vi "Main.vi"(11 "Module Admin":refnum<class "Delacor_lib_QMH_Cloneable Module Admin.lvclass">) -> ()   [LabVIEW 2024, in "cameraV1.lvlib"]
doc: "This template is based off of the Queued Message Handler design pattern and the Queued Message Handler project template that ships with LabVIEW.\n\nThe main difference is that the queue is private to this module and communication between modules is performed via Broadcast and Request events.\n\nRequest events are wrapped in public API methods and are handled in the Event Handling Loop (EHL) of this VI. Any module can register for Broadcast events sent by this module. The EHL generates messages based on user interface actions.\n\nThe Message Handling Loop (MHL) processes messages generated by the EHL, or by other messages. The messages are string values, so new messages can be added easily to the Message Cases case structure in the MHL. Each message cluster can also provide an optional value for Message Data, which is a variant that can be converted to whatever message-specific data is required.\n_____\nBased on DQMH Dev Tools: Project Template 7.1.0.1503."
uses:
  cameraV1.lvlib
  <vilib>/Delacor/Delacor QMH/Libraries/Cloneable Module Admin_class/Delacor_lib_QMH_Cloneable Module Admin.lvclass
  Controls/camera module state.ctl
  Controls/state.ctl
  Module Data--cluster.ctl
  <vilib>/Delacor/Delacor QMH/Libraries/Message Queue_class/Delacor_lib_QMH_Message Queue.lvclass/Delacor_lib_QMH_Message Queue.ctl
  <vilib>/Delacor/Delacor QMH/Libraries/Cloneable Module Admin_class/Delacor_lib_QMH_Cloneable Module Admin.lvclass/Delacor_lib_QMH_Cloneable Module Admin.ctl
  Stop Argument--cluster.ctl
  <vilib>/Delacor/Delacor QMH/Libraries/Module Admin_class/Delacor_lib_QMH_Module Admin.lvclass/Delacor_lib_QMH_Module Admin.ctl
  connect Argument--cluster.ctl
  Send_Command Argument--cluster.ctl
  Controls/commands 1.ctl
  Send_Command (Reply Payload)--cluster.ctl
  Cam Image Response Argument--cluster.ctl
  <vilib>/Utility/miscctls.llb/LVPointTypeDef.ctl
  <vilib>/Delacor/Delacor QMH/Libraries/Message Queue_class/Delacor_lib_QMH_Enqueue Message (Single).vi
  <vilib>/Delacor/Delacor QMH/Libraries/Cloneable Module Admin_class/Delacor_lib_QMH_Get Module ID.vi
  <vilib>/Delacor/Delacor QMH/Libraries/Module Admin_class/Delacor_lib_QMH_Get External Launch.vi
  <vilib>/Delacor/Delacor QMH/Libraries/Message Queue_class/Delacor_lib_QMH_Message Queue.lvclass
panel:
  out "serial":string
  out "error out":errorcluster
  out "Status":string
  in  "Simulate EHL Error":bool
  in  "Simulate MHL Error":bool
  # "Other processes communicate with this Module via its Public API (wrappers for its Request Events).\n\nThis Module communicates with other processes via its Broadcast Events.\nAny process that wants to receive these messages can register for this module's Broadcast events."
  # "This template is for the DQMH framework. See the block diagram for more information on how to use this template."
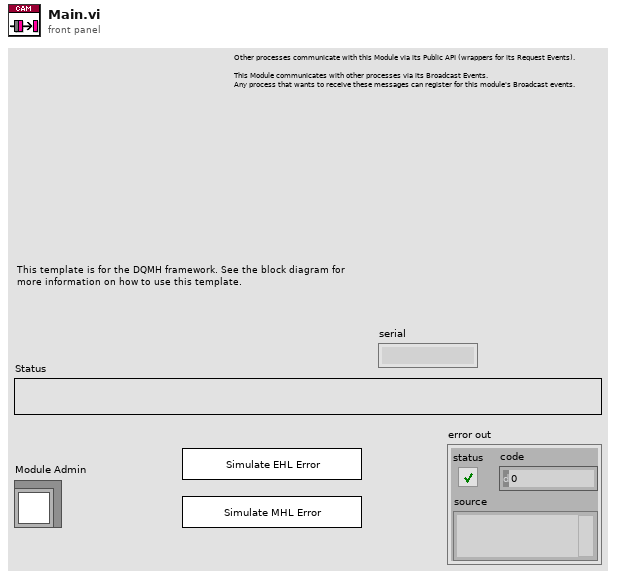
[diagram p1: front panel]
types:
  T1 = typedef "cameraV1.lvlib/camera module state.ctl" = cluster{"state":T2, "variant":variant}
  T2 = typedef "cameraV1.lvlib/state.ctl" = enum16{"connected", "not connected", "Online", "Offline"}
  T3 = typedef "cameraV1.lvlib/Request Events--cluster.ctl" = cluster{"Stop Module":refnum<user-event>, "Show Panel":refnum<user-event>, "Hide Panel":refnum<user-event>, "Show Diagram":refnum<user-event>, "Get Module Execution Status":refnum<user-event>, "connect":refnum<user-event>, "Send_Command":refnum<user-event>, "Cam Image Response":refnum<user-event>}
  T4 = typedef "cameraV1.lvlib/Module Data--cluster.ctl" = cluster{"Status":string, "send ID":refnum<k5>, "recived ID":refnum<k5>, "R_port_Status":bool, "S_port_Status":bool}
  T5 = enum32{"invalid lock state", "Not Locked", "Locked (No Password)", "Password-protected"}
  T6 = typedef "cameraV1.lvlib/Stop Argument--cluster.ctl" = cluster{"Module ID":i32, "Origin":string, "Exit via Stop Module Req?":bool, "Wait for Module to stop?":bool}
  T7 = typedef "cameraV1.lvlib/connect Argument--cluster.ctl" = cluster{"Module ID":i32, "ip":string, "R_port":dbl, "S_port":dbl, "timeout":dbl}
  T8 = typedef "cameraV1.lvlib/Send_Command Argument--cluster.ctl" = cluster{"Module ID":i32, "command":T9, "String":string, "Wait Notifier":refnum<notifier>, "wait for reply":bool, "Value":string, "Var Name":string}
  T9 = typedef "commands 1.ctl" = string
  T10 = typedef "cameraV1.lvlib/Cam Image Response Argument--cluster.ctl" = cluster{"Module ID":i32, "Boolean":bool}
  T11 = typedef "LVPointTypeDef.ctl" = cluster{"Horizontal":i16, "Vertical":i16}
  T12 = enum32{"Invalid", "Standard", "Closed", "Hidden", "Minimized", "Maximized"}
  T13 = typedef "cameraV1.lvlib/Send_Command (Reply Payload)--cluster.ctl" = cluster{"Module ID":i32, "Sucsses?":bool, "error":errorcluster}
  T14 = typedef "cameraV1.lvlib/commands 1.ctl" = string
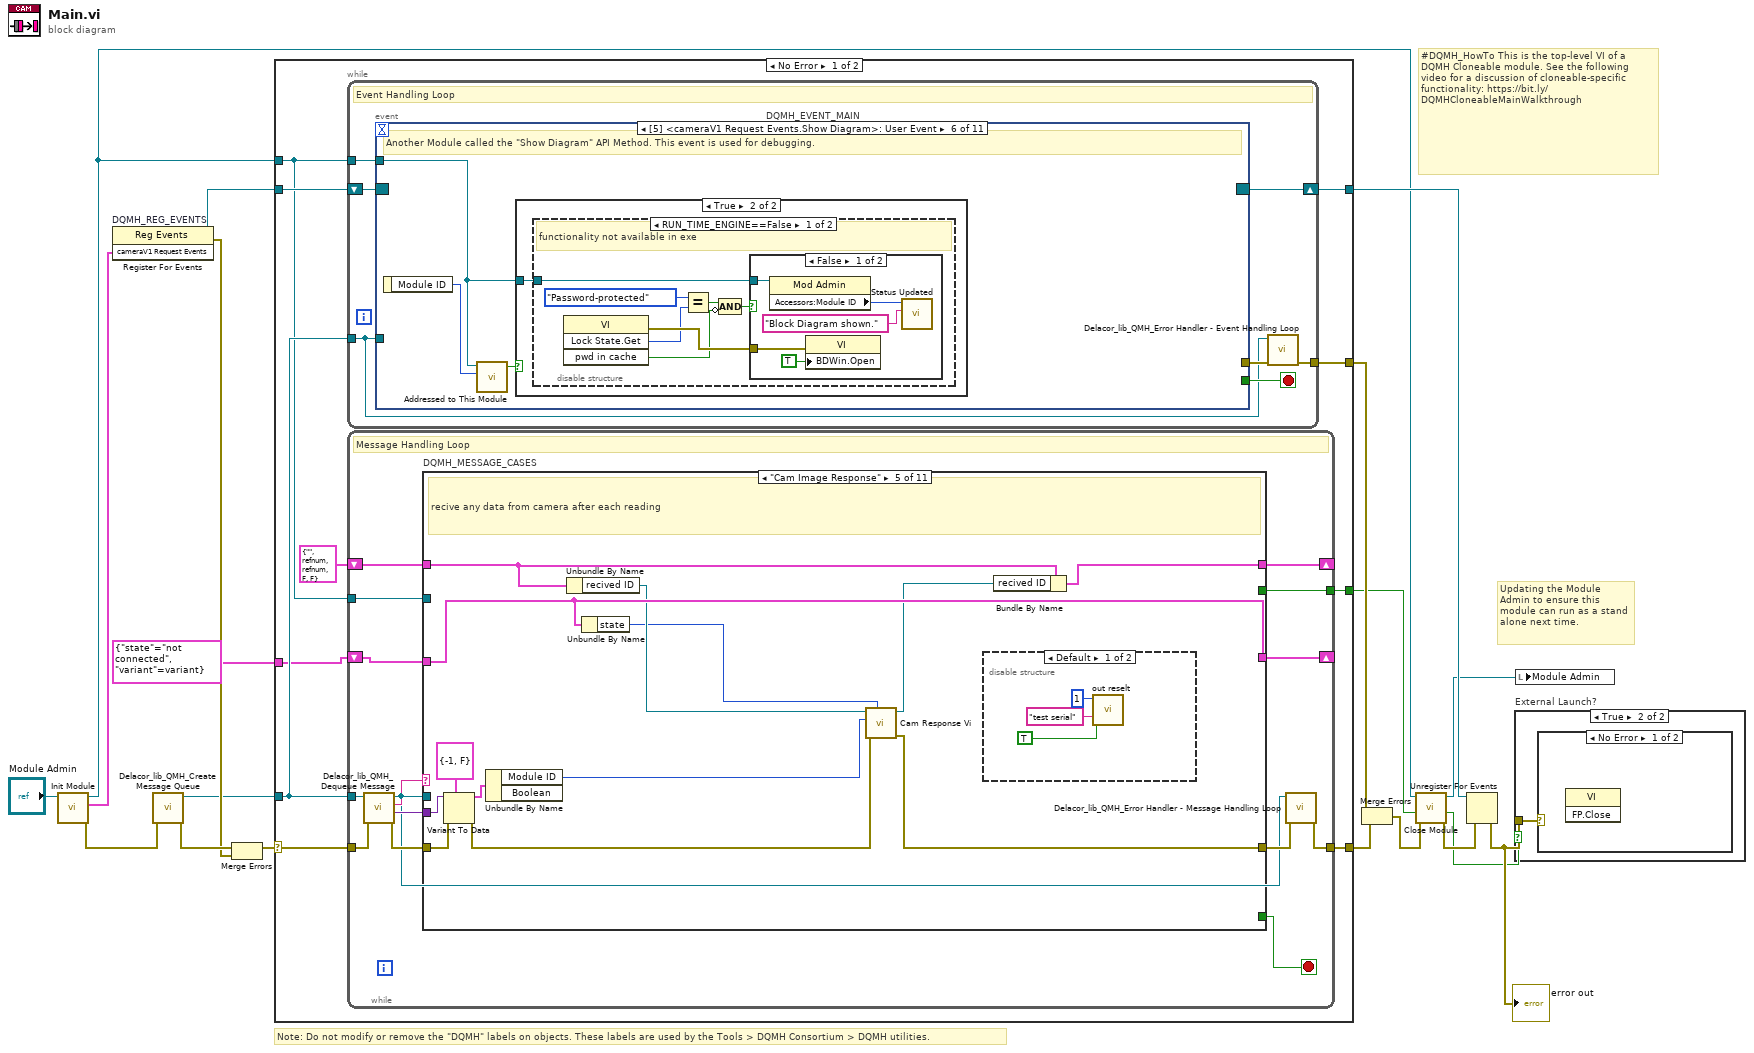
[diagram p0: block diagram]
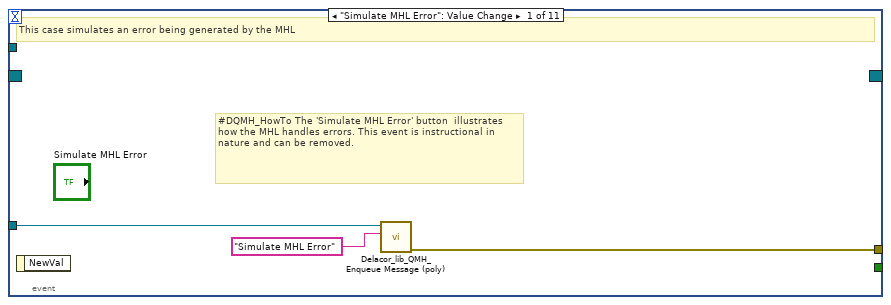
[diagram p2: hidden frame]
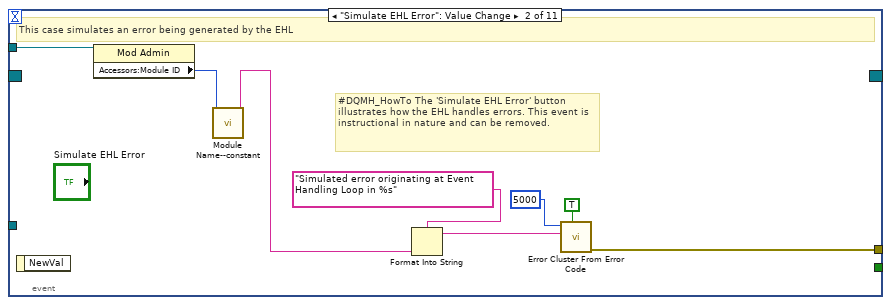
[diagram p3: hidden frame]
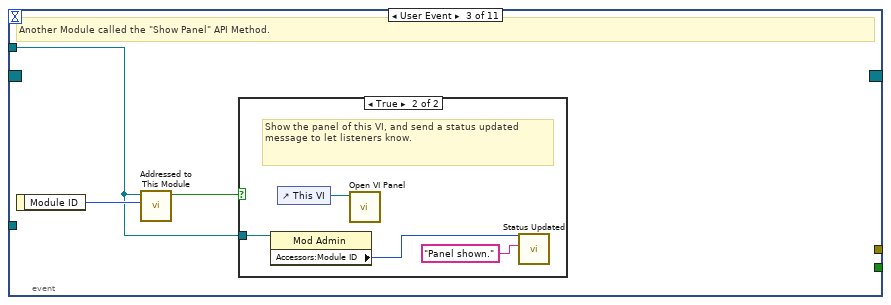
[diagram p4: hidden frame]
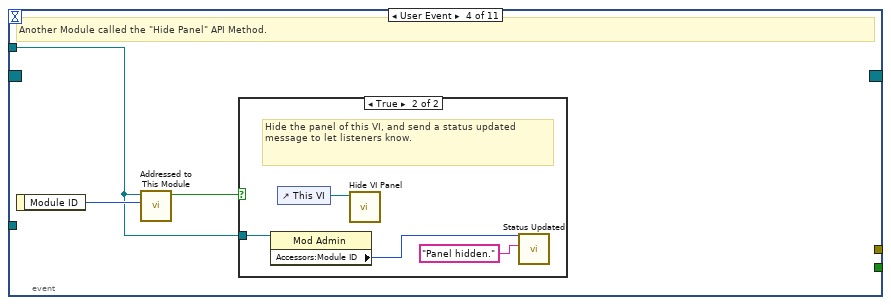
[diagram p6: hidden frame]
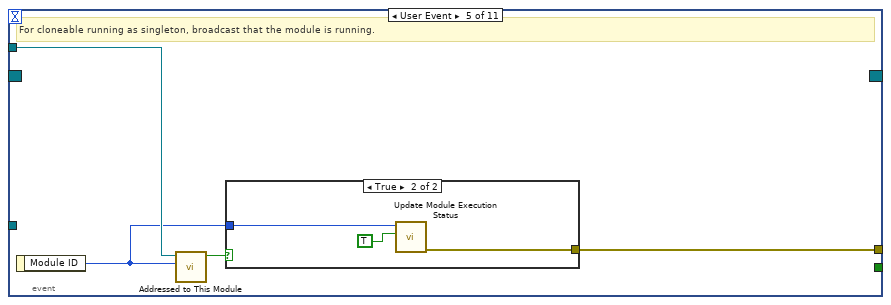
[diagram p8: hidden frame]
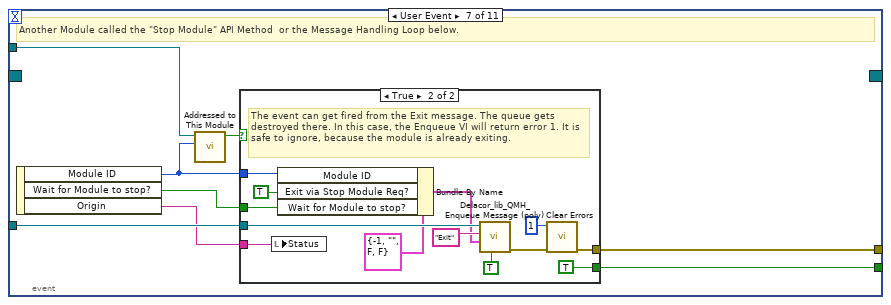
[diagram p13: hidden frame]
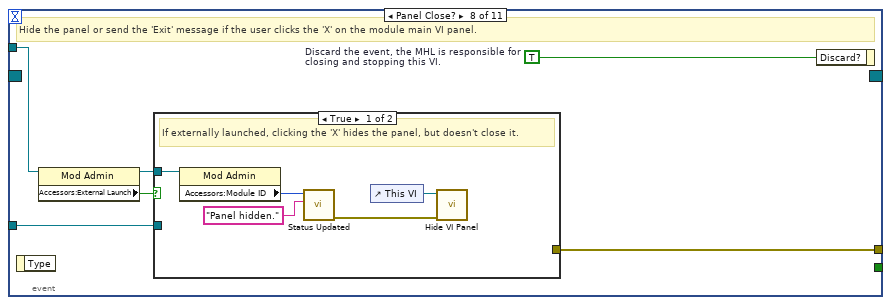
[diagram p15: hidden frame]
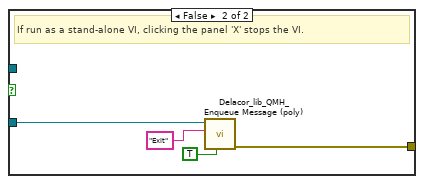
[diagram p16: hidden frame]
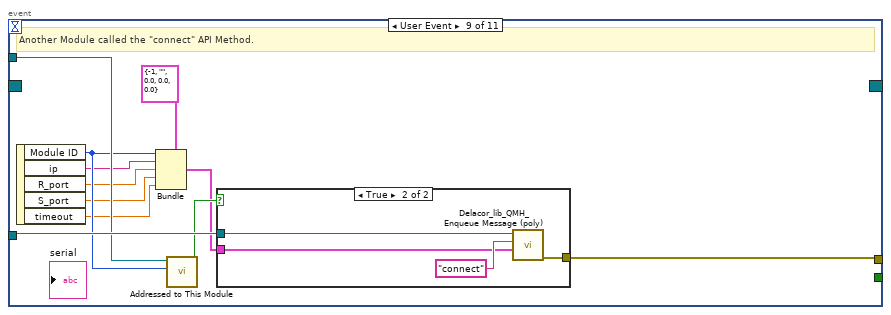
[diagram p17: hidden frame]
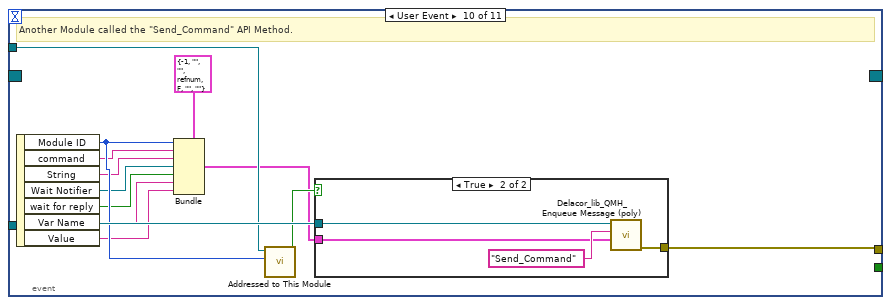
[diagram p19: hidden frame]
diagram:
  # "#DQMH_HowTo This is the top-level VI of a DQMH Cloneable module. See the following video for a discussion of cloneable-specific functionality: https://bit.ly/DQMHCloneableMainWalkthrough"
  # "Note: Do not modify or remove the \"DQMH\" labels on objects. These labels are used by the Tools > DQMH Consortium > DQMH utilities."
  # "Updating the Module Admin to ensure this module can run as a stand alone next time."
  n1 = call "Init Module.vi"("Cloneable Module Admin in"="Module Admin") -> ("error out"=w16:errorcluster, "cameraV1 Request Events"=w8:T3, "Cloneable Module Admin out"=w5:refnum<class "Delacor_lib_QMH_Cloneable Module Admin.lvclass">)  [unwired: 8 in]
  n2 = register-events "DQMH_REG_EVENTS"(w8) -> (reference out=w9:refnum<event-registration>, error out=w11:errorcluster)  [unwired: 2 in]
  n3 = call <vilib>:"Delacor_lib_QMH_Create Message Queue.vi"("error in"=w16) -> ("error out"=w13:errorcluster, "Message Queue"=w7:refnum<class "Delacor_lib_QMH_Message Queue.lvclass">)  [unwired: 9 in]
  n4 = Merge Errors(w13, w11) -> (w12:errorcluster)
  n5 = case shown="No Error" w12 {
    selector: w12 -> [w27 w362]
    tunnel: [w29 w361] -> w17
    tunnel: [w26 w360] -> w10
    tunnel: w9 -> [w24 w360]
    tunnel: w7 -> [w23 w353]
    tunnel: [w28 _] -> w18
    tunnel: w5 -> [w22 w356]
    tunnel: [w21 _] -> w3
    tunnel: T1 {"state"=enum."not connected", "variant"=variant} -> [w20 _]
    frame No Error {
      n6 = while {
        tunnel: w23 -> [w30]
        shift-right: [w33] -> w26
        shift-left: w24 -> [w34]
        tunnel: [w35] -> w28
        tunnel: w22 -> [w31]
        stop <- w32 stop-if-true
        # "Event Handling Loop"
        n7 = event "DQMH_EVENT_MAIN" shown="[5] <cameraV1 Request Events.Show Diagram>: User Event" {
          selector: w34 -> [_ _ _ _ _ _ _ _ _ _ _]
          dyn-events: [_ _ _ _ _ _ _ _ _ _ _] -> w33
          timeout: _ -> [_ _ _ _ _ _ _ _ _ _ _]
          tunnel: [_ _ _ _ _ _ w88 _ _ _ _] -> w32
          tunnel: w30 -> [w38 _ _ _ _ _ w91 w108 w131 w148 w160]
          tunnel: [w39 w47 _ _ w65 _ w92 w111 w123 w138 w153] -> w36
          tunnel: w31 -> [_ w46 w48 w55 w63 w69 w90 w109 w129 w146 w158]
          event "Simulate MHL Error": Value Change {
            # "#DQMH_HowTo The 'Simulate MHL Error' button  illustrates how the MHL handles errors. This event is instructional in nature and can be removed."
            # "This case simulates an error being generated by the MHL"
            n8 = event-data() -> ()  [unwired: 1 in, 1 out]
            n9 = call-poly <vilib>:"Delacor_lib_QMH_Enqueue Message (poly).vi"("Message"="Simulate MHL Error", "Message Queue in"=w38) -> ("error out"=w39:errorcluster)  [unwired: 8 in, 1 out]
          }
          event "Simulate EHL Error": Value Change {
            # "#DQMH_HowTo The 'Simulate EHL Error' button  illustrates how the EHL handles errors. This event is instructional in nature and can be removed."
            # "This case simulates an error being generated by the EHL"
            n10 = event-data() -> ()  [unwired: 1 in, 1 out]
            n11 = property on="Property Node" class="Mod Admin"(reference=w46) -> ("Accessors:Module ID"=w45:i32)  [unwired: 1 in, 2 out]
            n12 = call "Module Name--constant.vi"("Module ID"=w45) -> ("Module Name"=w40:string)  [unwired: 10 in]
            n13 = Format Into String(format string="Simulated error originating at Event Handling Loop in %s", w40) -> (resulting string=w43:string)  [unwired: 2 in, 1 out]
            n14 = call <vilib>:"Error Cluster From Error Code.vi"("show call chain? (False)"=TRUE, "error message (\"\")"=w43, "error code (0)"=5000) -> ("error out"=w47:errorcluster)  [unwired: 6 in]
          }
          event User Event {
            # "Another Module called the \"Show Panel\" API Method."
            n15 = event-data() -> ("Module ID"=w49:i32)  [unwired: 1 in]
            n16 = call "Addressed to This Module.vi"("Module ID from Argument"=w49, "Module Admin"=w48) -> ("Addressed to this instance?"=w50:bool)  [unwired: 8 in, 1 out]
            n17 = case shown="True" w50 {
              tunnel: w48 -> [_ w52]
              frame False {
              }
              frame True {
                # "Show the panel of this VI, and send a status updated message to let listeners know."
                n18 = property on="Property Node" class="Mod Admin"(reference=w52) -> ("Accessors:Module ID"=w51:i32)  [unwired: 1 in, 2 out]
                n19 = control-ref of="This VI"() -> (w54:refnum<vi>)
                n20 = call "Open VI Panel.vi"("VI"=w54) -> ()  [unwired: 10 in, 1 out]
                n21 = call "Status Updated.vi"("Status"="Panel shown." ("format string"), "Module ID"=w51) -> ()  [unwired: 9 in, 1 out]
              }
            }
          }
          event User Event {
            # "Another Module called the \"Hide Panel\" API Method."
            n22 = event-data() -> ("Module ID"=w56:i32)  [unwired: 1 in]
            n23 = call "Addressed to This Module.vi"("Module ID from Argument"=w56, "Module Admin"=w55) -> ("Addressed to this instance?"=w57:bool)  [unwired: 8 in, 1 out]
            n24 = case shown="True" w57 {
              tunnel: w55 -> [_ w59]
              frame False {
              }
              frame True {
                # "Hide the panel of this VI, and send a status updated message to let listeners know."
                n25 = property on="Property Node" class="Mod Admin"(reference=w59) -> ("Accessors:Module ID"=w58:i32)  [unwired: 1 in, 2 out]
                n26 = control-ref of="This VI"() -> (w61:refnum<vi>)
                n27 = call "Hide VI Panel.vi"("VI"=w61) -> ()  [unwired: 10 in, 1 out]
                n28 = call "Status Updated.vi"("Status"="Panel hidden." ("format string"), "Module ID"=w58) -> ()  [unwired: 9 in, 1 out]
              }
            }
          }
          event User Event {
            # "For cloneable running as singleton, broadcast that the module is running."
            n29 = event-data() -> ("Module ID"=w62:i32)  [unwired: 1 in]
            n30 = call "Addressed to This Module.vi"("Module ID from Argument"=w62, "Module Admin"=w63) -> ("Addressed to this instance?"=w64:bool)  [unwired: 8 in, 1 out]
            n31 = case shown="True" w64 {
              tunnel: [_ w68] -> w65
              tunnel: w62 -> [_ w67]
              frame False {
              }
              frame True {
                n32 = call "Update Module Execution Status.vi"("Running?"=TRUE, "Module ID"=w67) -> ("error out"=w68:errorcluster)  [unwired: 9 in]
              }
            }
          }
          event User Event {
            # "Another Module called the \"Show Diagram\" API Method. This event is used for debugging."
            n33 = event-data() -> ("Module ID"=w70:i32)  [unwired: 1 in]
            n34 = call "Addressed to This Module.vi"("Module ID from Argument"=w70, "Module Admin"=w69) -> ("Addressed to this instance?"=w71:bool)  [unwired: 8 in, 1 out]
            n35 = case shown="True" w71 {
              tunnel: w69 -> [_ w72]
              frame False {
              }
              frame True {
                n36 = disable-structure shown="RUN_TIME_ENGINE==False" {
                  disable-tunnel: w72 -> [w73 _]
                  frame condition #0 (active) {
                    # "functionality not available in exe"
                    n37 = invoke on="Invoke Node" class="VI" method="Lock State.Get"() -> (error out=w79:errorcluster, "Get Lock State"=w78:T5, "pwd in cache"=w75:bool)  [unwired: 4 in, 1 out]
                    n38 = Equal?(x=T5."Password-protected", y=w78) -> (x = y?=w76:bool)
                    n39 = Compound Arithmetic op=AND(w76, invert w75) -> (w74:bool)
                    n40 = case shown="False" w74 {
                      tunnel: w79 -> [w84 _]
                      tunnel: w73 -> [w81 _]
                      frame False {
                        n41 = property on="Property Node" class="Mod Admin"(reference=w81) -> ("Accessors:Module ID"=w80:i32)  [unwired: 1 in, 2 out]
                        n42 = property on="Property Node" class="VI"(error in=w84, "BDWin.Open"=TRUE ("Block Diagram Window:Open")) -> ()  [unwired: 1 in, 2 out]
                        n43 = call "Status Updated.vi"("Status"="Block Diagram shown." ("format string"), "Module ID"=w80) -> ()  [unwired: 9 in, 1 out]
                      }
                      frame True {
                        # "Password-protected VI, and the password is not in the cache. Do not show the diagram."
                      }
                    }
                  }
                  frame condition #1 {
                  }
                }
              }
            }
          }
          event User Event {
            # "Another Module called the \"Stop Module\" API Method  or the Message Handling Loop below."
            n44 = event-data() -> ("Module ID"=w86:i32, "Wait for Module to stop?"=w87:bool, "Origin"=w85:string)  [unwired: 1 in]
            n45 = call "Addressed to This Module.vi"("Module ID from Argument"=w86, "Module Admin"=w90) -> ("Addressed to this instance?"=w89:bool)  [unwired: 8 in, 1 out]
            n46 = case shown="True" w89 {
              tunnel: [_ w104] -> w92
              tunnel: w91 -> [_ w100]
              tunnel: [_ TRUE] -> w88
              tunnel: w87 -> [_ w95]
              tunnel: w86 -> [_ w97]
              tunnel: w85 -> [_ w93]
              frame False {
              }
              frame True {
                # "The event can get fired from the Exit message. The queue gets destroyed there. In this case, the Enqueue VI will return error 1. It is safe to ignore, because the module is already exiting."
                n47 = local write "Status"(w93) -> ()
                n48 = Bundle By Name(cluster=T6 {"Module ID"=-1, "Origin"="", "Exit via Stop Module Req?"=FALSE, "Wait for Module to stop?"=FALSE} ("Stop Argument"), "Module ID"=w97, "Exit via Stop Module Req?"=TRUE, "Wait for Module to stop?"=w95) -> (w94:T6)
                n49 = call-poly <vilib>:"Delacor_lib_QMH_Enqueue Message (poly).vi"("Priority Message? (F)"=TRUE, "Message Data"=w94, "Message"="Exit", "Message Queue in"=w100) -> ("error out"=w105:errorcluster)  [unwired: 6 in, 1 out]
                n50 = call <vilib>:"Clear Errors.vi"("error in (no error)"=w105, "specific error code to clear (0: all)"=1) -> ("error out"=w104:errorcluster)  [unwired: 4 in, 1 out]
              }
            }
          }
          event Panel Close? {
            w110 = TRUE  # Discard the event, the MHL is responsible for closing and stopping this VI.
            # "Hide the panel or send the 'Exit' message if the user clicks the 'X' on the module main VI panel."
            n51 = event-data() -> ()  [unwired: 1 in, 1 out]
            n52 = property on="Property Node" class="Mod Admin"(reference=w109) -> (reference out=w106:refnum<class "Delacor_lib_QMH_Cloneable Module Admin.lvclass">, "Accessors:External Launch"=w107:bool)  [unwired: 1 in, 1 out]
            n53 = case shown="True" w107 {
              tunnel: w108 -> [_ w119]
              tunnel: [_ w120] -> w111
              tunnel: w106 -> [w114 _]
              frame True {
                # "If externally launched, clicking the 'X' hides the panel, but doesn't close it."
                n54 = property on="Property Node" class="Mod Admin"(reference=w114) -> ("Accessors:Module ID"=w113:i32)  [unwired: 1 in, 2 out]
                n55 = call "Status Updated.vi"("Status"="Panel hidden." ("format string"), "Module ID"=w113) -> ("error out"=w112:errorcluster)  [unwired: 9 in]
                n56 = control-ref of="This VI"() -> (w116:refnum<vi>)
                n57 = call "Hide VI Panel.vi"("error in"=w112, "VI"=w116) -> ()  [unwired: 9 in, 1 out]
              }
              frame False {
                # "If run as a stand-alone VI, clicking the panel 'X' stops the VI."
                n58 = call-poly <vilib>:"Delacor_lib_QMH_Enqueue Message (poly).vi"("Priority Message? (F)"=TRUE, "Message"="Exit", "Message Queue in"=w119) -> ("error out"=w120:errorcluster)  [unwired: 7 in, 1 out]
              }
            }
            n59 = event-data ("Event Filter Node")("Discard?"=w110) -> ()  [unwired: 1 in, 1 out]
          }
          event User Event {
            # "Another Module called the \"connect\" API Method."
            n60 = event-data() -> ("Module ID"=w126:i32, "ip"=w125:string, "R_port"=w124:dbl, "S_port"=w122:dbl, "timeout"=w121:dbl)  [unwired: 1 in]
            n61 = Bundle(cluster=T7 {"Module ID"=-1, "ip"="", "R_port"=0.0, "S_port"=0.0, "timeout"=0.0} ("connect Argument"), "Module ID"=w126, "ip"=w125, "R_port"=w124, "S_port"=w122, "timeout"=w121) -> (w127:T7)
            n62 = call "Addressed to This Module.vi"("Module ID from Argument"=w126, "Module Admin"=w129) -> ("Addressed to this instance?"=w130:bool)  [unwired: 8 in, 1 out]
            n63 = case shown="True" w130 {
              tunnel: w131 -> [_ w135]
              tunnel: w127 -> [_ w133]
              tunnel: [_ w132] -> w123
              frame False {
              }
              frame True {
                n64 = call-poly <vilib>:"Delacor_lib_QMH_Enqueue Message (poly).vi"("Message Data"=w133, "Message"="connect", "Message Queue in"=w135) -> ("error out"=w132:errorcluster)  [unwired: 7 in, 1 out]
              }
            }
          }
          event User Event {
            # "Another Module called the \"Send_Command\" API Method."
            n65 = event-data() -> ("Module ID"=w143:i32, "command"=w142:T14, "String"=w141:string, "Wait Notifier"=w140:refnum<notifier>, "wait for reply"=w139:bool, "Var Name"=w137:string, "Value"=w136:string)  [unwired: 1 in]
            n66 = Bundle(cluster=T8 {"Module ID"=-1, "command"="", "String"="", "Wait Notifier"=refnum, "wait for reply"=FALSE, "Value"="", "Var Name"=""} ("Send_Command Argument"), "Module ID"=w143, "command"=w142, "String"=w141, "Wait Notifier"=w140, "wait for reply"=w139, "Value"=w137, "Var Name"=w136) -> (w144:T8)
            n67 = call "Addressed to This Module.vi"("Module ID from Argument"=w143, "Module Admin"=w146) -> ("Addressed to this instance?"=w147:bool)  [unwired: 8 in, 1 out]
            n68 = case shown="True" w147 {
              tunnel: w148 -> [_ w152]
              tunnel: w144 -> [_ w150]
              tunnel: [_ w149] -> w138
              frame False {
              }
              frame True {
                n69 = call-poly <vilib>:"Delacor_lib_QMH_Enqueue Message (poly).vi"("Message Data"=w150, "Message"="Send_Command", "Message Queue in"=w152) -> ("error out"=w149:errorcluster)  [unwired: 7 in, 1 out]
              }
            }
          }
          event User Event {
            # "Another Module called the \"Cam Image Response\" API Method."
            n70 = event-data() -> ("Module ID"=w155:i32, "Boolean"=w154:bool)  [unwired: 1 in]
            n71 = Bundle(cluster=T10 {"Module ID"=-1, "Boolean"=FALSE} ("Cam Image Response Argument"), "Module ID"=w155, "Boolean"=w154) -> (w156:T10)
            n72 = call "Addressed to This Module.vi"("Module ID from Argument"=w155, "Module Admin"=w158) -> ("Addressed to this instance?"=w159:bool)  [unwired: 8 in, 1 out]
            n73 = case shown="True" w159 {
              tunnel: w160 -> [_ w164]
              tunnel: w156 -> [_ w162]
              tunnel: [_ w161] -> w153
              frame False {
              }
              frame True {
                n74 = call-poly <vilib>:"Delacor_lib_QMH_Enqueue Message (poly).vi"("Message Data"=w162, "Message"="Cam Image Response", "Message Queue in"=w164) -> ("error out"=w161:errorcluster)  [unwired: 7 in, 1 out]
              }
            }
          }
        }
        n75 = call-dynamic "Delacor_lib_QMH_Error Handler - Event Handling Loop.vi"("error in"=w36, "Message Queue in"=w30) -> ("dup error in"=w35:errorcluster)  [unwired: 8 in, 1 out]
      }
      n76 = while {
        tunnel: w23 -> [w167]
        shift-right: [w174] -> _
        shift-left: T4 {"Status"="", "send ID"=refnum, "recived ID"=refnum, "R_port_Status"=FALSE, "S_port_Status"=FALSE} ("Data Cluster") -> [w175]
        tunnel: w27 -> [w178]
        tunnel: [w176] -> w29
        tunnel: w22 -> [w169]
        tunnel: [w168] -> w21
        shift-right: [w165] -> _
        shift-left: w20 -> [w166]
        stop <- w173 stop-if-true
        # "Message Handling Loop"
        n77 = call-dynamic "Delacor_lib_QMH_Dequeue Message.vi"("error in"=w178, "Message Queue in"=w167) -> ("error out"=w177:errorcluster, "Message Data"=w171:variant, "Message"=w172:string, "Message Queue out"=w170:refnum<class "Delacor_lib_QMH_Message Queue.lvclass">)  [unwired: 6 in]
        n78 = case "DQMH_MESSAGE_CASES" shown="\"Cam Image Response\"" w172 {
          selector: w172 -> [_ _ _ _ _ _ _ _ _ _ w342]
          tunnel: w170 -> [_ _ _ _ _ _ _ w294 _ w333 _]
          tunnel: w177 -> [w199 w204 w225 w260 w280 w287 w290 w303 w321 w339 w351]
          tunnel: [w197 w204 w211 w242 w269 w286 w290 w299 w320 w334 w352] -> w179
          tunnel: w175 -> [w190 w203 w218 w246 w275 w285 w289 w298 w318 w332 w349]
          tunnel: [w189 w203 w217 w245 w274 w285 w289 w298 w318 w332 w349] -> w174
          tunnel: [_ _ _ _ _ _ _ _ _ w331 _] -> w173
          tunnel: w171 -> [_ _ w224 w259 w279 _ _ w297 _ w329 _]
          tunnel: w169 -> [w185 _ _ w251 _ _ _ w296 w316 w324 w348]
          tunnel: [_ _ _ _ _ _ _ _ _ w327 _] -> w168
          tunnel: w166 -> [w180 w202 w205 w236 w276 w284 w288 w291 w310 w322 w340]
          tunnel: [w180 w202 w205 w235 w276 w284 w288 w291 w310 w322 w340] -> w165
          frame "Initialize" {
            w182 = "Initial Message" ("Initial Message")
            # "#DQMH_CodeNeeded - Initialize the appearance of the front panel."
            # "#DQMH_CodeNeeded - Initialize your state data here."
            # "Initialize - Any operation that needs to be done before the module can receive messages. Synchronize Caller Events.vi will inform Start Module.vi that the module has launched and is ready to receive messages. Module Did Init.vi will broadcast that the module initialized."
            n79 = call "Synchronize Caller Events.vi"("error in"=w199, "Module Admin"=w185) -> ("error out"=w198:errorcluster, "Module Admin out"=w184:refnum<class "Delacor_lib_QMH_Cloneable Module Admin.lvclass">)  [unwired: 8 in]
            n80 = property on="Property Node" class="Mod Admin"(reference=w184) -> ("Accessors:Module ID"=w181:i32, "Accessors:External Launch"=w186:bool)  [unwired: 1 in, 2 out]
            n81 = call "Module Name--constant.vi"("Module ID"=w181) -> ("Module Name"=w194:string)  [unwired: 10 in]
            n82 = property on="Property Node" class="VI"("Front Panel.Title"=w194) -> (reference out=w196:refnum<vi>, error out=w201:errorcluster)  [unwired: 2 in]
            n83 = Select(t=T12."Hidden" ("State"), s=w186, f=T12."Standard" ("State")) -> (s? t:f=w191:T12)
            n84 = invoke on="Invoke Node" class="VI" method="FP.Open"(reference=w196, error in=w201, "State"=w191) -> (reference out=w195:refnum<vi>, error out=w200:errorcluster)  [unwired: 2 in, 3 out]
            n85 = Bundle By Name(cluster=w190, "Status"=w182) -> (w189:T4)
            n86 = invoke on="Invoke Node" class="VI" method="FP.Center"(reference=w195, error in=w200) -> ()  [unwired: 1 in, 3 out]
            n87 = property on="Pane" class="Pane"("Origin"=T11 {"Horizontal"=0, "Vertical"=0}) -> ()  [unwired: 2 in, 2 out]
            n88 = call "Module Name--constant.vi"("Module ID"=w181) -> ("Module Name"=w187:string)  [unwired: 10 in]
            n89 = call "Module Did Init.vi"("error in"=w198, "Initialized?"=TRUE, "Origin"=w187, "Module ID"=w181) -> ("error out"=w197:errorcluster)  [unwired: 7 in]
            "Status" <- w182
          }
          frame "---Module Specific---" {
            # "Separator -- The following cases handle messages specific to this Module."
          }
          frame "connect" {
            n90 = Variant To Data(error in=w225, type=T7 {"Module ID"=-1, "ip"="", "R_port"=0.0, "S_port"=0.0, "timeout"=0.0} ("connect Argument"), Variant=w224) -> (data=w222:T7, error out=w212:errorcluster)
            n91 = Unbundle By Name(w222) -> ("ip"=w220:string, "R_port"=w221:dbl, "S_port"=w219:dbl, "timeout"=w208:dbl)  [unwired: 1 out]
            n92 = TCP Open Connection(address=w220, remote port or service name=w221, timeout ms (60000)=w208, error in (no error)=w212) -> (connection ID=w216:refnum<k5>, error out=w214:errorcluster)  [unwired: 1 in]
            n93 = TCP Open Connection(address=w220, remote port or service name=w219, timeout ms (60000)=w208, error in (no error)=w212) -> (connection ID=w215:refnum<k5>, error out=w213:errorcluster)  [unwired: 1 in]
            n94 = case shown="No Error" w214 {
              selector: w214 -> [w231 w233]
              tunnel: [w231 w233] -> w209
              tunnel: [TRUE FALSE] -> w207
              frame No Error {
              }
              frame Error {
              }
            }
            n95 = case shown="No Error" w213 {
              selector: w213 -> [w227 w229]
              tunnel: [w227 w229] -> w210
              tunnel: [TRUE FALSE] -> w206
              frame No Error {
              }
              frame Error {
              }
            }
            n96 = Merge Errors(w209, w210) -> (w211:errorcluster)
            n97 = Bundle By Name(cluster=w218, "recived ID"=w216, "send ID"=w215, "R_port_Status"=w207, "S_port_Status"=w206) -> (w217:T4)
          }
          frame "Send_Command" {
            # "send any command to cam ex load project , get status, send variable"
            n98 = property class="Mod Admin"(reference=w251) -> ("Accessors:Module ID"=w252:i32)  [unwired: 1 in, 2 out]
            n99 = Variant To Data(error in=w260, type=T8 {"Module ID"=-1, "command"="", "String"="", "Wait Notifier"=refnum, "wait for reply"=FALSE, "Value"="", "Var Name"=""} ("Send_Command Argument"), Variant=w259) -> (data=w257:T8, error out=w243:errorcluster)
            n100 = Unbundle By Name(w257) -> ("Module ID"=w234:i32, "command"=w240:T9, "String"=w249:string, "Var Name"=w248:string, "Value"=w247:string, "Wait Notifier"=w256:refnum<notifier>, "wait for reply"=w255:bool)
            n101 = Unbundle By Name(w246) -> ("send ID"=w250:refnum<k5>)
            n102 = Equal?(x=w240, y="StartMode") -> (x = y?=w237:bool)
            n103 = call "Camera Command Handle.vi"("Value"=w247, "Var Name"=w248, "error in (no error)"=w243, "String"=w249, "command"=w240, "connection ID"=w250) -> ("error out"=w242:errorcluster, "Command Accepted"=w238:bool, "connection ID 2"=w244:refnum<k5>)  [unwired: 3 in]
            n104 = And(x=w238, y=w237) -> (x .and. y?=w239:bool)
            n105 = case shown="True" w239 {
              tunnel: w236 -> [w261 w265]
              tunnel: [w261 w263] -> w235
              tunnel: w234 -> [_ w262]
              frame False {
              }
              frame True {
                n106 = call "Cam Image Response.vi"("Module ID"=w262) -> ()  [unwired: 10 in, 1 out]
                n107 = Bundle By Name(cluster=w265, "state"=state."Online") -> (w263:T1)
              }
            }
            n108 = Bundle By Name(cluster=w246, "send ID"=w244) -> (w245:T4)
            n109 = Bundle By Name(cluster=T13 {"Module ID"=-1, "Sucsses?"=FALSE, "error"={"status"=FALSE, "code"=0, "source"=""}} ("Send_Command (Reply Payload)"), "Module ID"=w252, "Sucsses?"=w238, "error"=w242) -> (w254:T13)
            n110 = case "DQMH_FIRE_NOTIFIER" shown="True" w255 {
              tunnel: w256 -> [_ w267]
              tunnel: w254 -> [_ w266]
              frame False {
              }
              frame True {
                n111 = Send Notification(notification=w266, notifier=w267) -> ()  [unwired: 1 in, 2 out]
              }
            }
          }
          frame "Cam Image Response" {
            # "recive any data from camera after each reading"
            n112 = Variant To Data(error in=w280, type=T10 {"Module ID"=-1, "Boolean"=FALSE} ("Cam Image Response Argument"), Variant=w279) -> (data=w277:T10, error out=w270:errorcluster)
            n113 = Unbundle By Name(w277) -> ("Module ID"=w272:i32)  [unwired: 1 out]
            n114 = Unbundle By Name(w275) -> ("recived ID"=w273:refnum<k5>)
            n115 = Unbundle By Name(w276) -> ("state"=w271:T2)
            n116 = call "Cam Response Vi.vi"("state"=w271, "error in"=w270, "Module ID"=w272, "recived ID"=w273) -> ("error out"=w269:errorcluster, "recived ID 2"=w268:refnum<k5>)  [unwired: 6 in]
            n117 = disable-structure shown="Default" {
              frame condition #0 (active) {
                n118 = call "out reselt.vi"("status"=TRUE, "serial"="test serial", "Module ID"=1) -> ()  [unwired: 8 in, 1 out]
              }
              frame condition #1 {
              }
            }
            n119 = Bundle By Name(cluster=w275, "recived ID"=w268) -> (w274:T4)
          }
          frame "---Copy This Frame---" {
            # "Duplicate this frame when creating new messages.  Change this comment in the duplicated frame to describe this message."
            n120 = Merge Errors(w287) -> (w286:errorcluster)
          }
          frame "---Exit and Error Handling---" {
            # "Separator - the following cases handle errors and exit messages."
          }
          frame "Error" {
            # "#DQMH_CodeRecommended - If the module is running in standalone mode (External Launch = FALSE), this code will pop up an error dialog and call the 'Exit' message if an error occurs. Add more fine-grained error management here."
            # "Error - Check the error message data and respond accordingly. This message is sent by the \"Error Handler\" VIs at the end of each loop in this application."
            n121 = property on="Property Node" class="Mod Admin"(reference=w296) -> ("Accessors:External Launch"=w295:bool, "Accessors:Module ID"=w293:i32)  [unwired: 1 in, 2 out]
            n122 = Variant To Data(error in=w303, type=errorcluster {"status"=FALSE, "code"=0, "source"=""} ("error constant"), Variant=w297) -> (data=w292:errorcluster, error out=w301:errorcluster)
            n123 = local write "error out"(w292) -> ()
            n124 = call "Error Reported.vi"("Error"=w292, "Module ID"=w293) -> ()  [unwired: 9 in, 1 out]
            n125 = case shown="False" w295 {
              tunnel: [w308 _] -> w300
              tunnel: w294 -> [w306 _]
              tunnel: w292 -> [w307 _]
              frame False {
                n126 = disable-structure shown="Default" {
                  disable-tunnel: w307 -> [w309 _]
                  frame condition #0 (active) {
                    # "If the module is running standalone, then pop up an error dialog and call the \"Exit\" message."
                    n127 = call <vilib>:"Simple Error Handler.vi"("error in (no error)"=w309) -> ()  [unwired: 4 in, 5 out]
                  }
                  frame condition #1 {
                    # "To prevent the Simple Error Handler VI from being loaded (e.g. when deploying to a Real-Time target), add the Conditional Disable Symbol \"DQMH_Disable_SEH\" to your project and set it to TRUE."
                  }
                }
                n128 = call-poly <vilib>:"Delacor_lib_QMH_Enqueue Message (poly).vi"("Priority Message? (F)"=TRUE, "Message"="Exit", "Message Queue in"=w306) -> ("error out"=w308:errorcluster)  [unwired: 7 in, 1 out]
              }
              frame True {
                # "If the module was launched externally, calling the Error Reported broadcast VI is the only action performed by the \"Error\" message. The module's caller can then process the error appropriately."
              }
            }
            n129 = Merge Errors(w301, w300) -> (w299:errorcluster)
          }
          frame "Simulate MHL Error" {
            # "#DQMH_HowTo The 'Simulate MHL Error' button  illustrates how the MHL handles errors. This event is instructional in nature and can be removed."
            # "Simulate an error occurring at the MHL"
            n130 = property on="Property Node" class="Mod Admin"(reference=w316) -> ("Accessors:Module ID"=w317:i32)  [unwired: 1 in, 2 out]
            n131 = call "Module Name--constant.vi"("Module ID"=w317) -> ("Module Name"=w312:string)  [unwired: 10 in]
            n132 = Format Into String(format string="Simulated error originating at Message Handling Loop in %s", w312) -> (resulting string=w313:string)  [unwired: 2 in, 1 out]
            n133 = call <vilib>:"Error Cluster From Error Code.vi"("show call chain? (False)"=TRUE, "error message (\"\")"=w313, "error code (0)"=5001) -> ("error out"=w319:errorcluster)  [unwired: 6 in]
            n134 = Merge Errors(w321, w319) -> (w320:errorcluster)
          }
          frame "Exit" {
            w330 = 91  # 91: not all Exit messages will have an argument
            w331 = TRUE  # Stop the VI
            # "Release the message queue reference"
            # "#DQMH_CodeNeeded - Add any required cleanup code here."
            # "Exit - Exit the application."
            n135 = Variant To Data(error in=w339, type=T6 {"Module ID"=-1, "Origin"="", "Exit via Stop Module Req?"=FALSE, "Wait for Module to stop?"=FALSE} ("Stop Argument"), Variant=w329) -> (data=w326:T6, error out=w335:errorcluster)
            n136 = call <vilib>:"Clear Errors.vi"("error in (no error)"=w335, "specific error code to clear (0: all)"=w330) -> ("error out"=w338:errorcluster)  [unwired: 4 in, 1 out]
            n137 = property on="Property Node" class="Mod Admin"(reference=w324) -> ("Accessors:Module ID"=w323:i32)  [unwired: 1 in, 2 out]
            n138 = control-ref of="This VI"() -> (w325:refnum<vi>)
            n139 = call-dynamic "Delacor_lib_QMH_Release Message Queue.vi"("error in"=w338, "Message Queue"=w333) -> ("error out"=w337:errorcluster)  [unwired: 9 in]
            n140 = call "Handle Exit.vi"("Stop Argument"=w326, "Module Admin in"=w324, "VI reference"=w325) -> ("error out"=w336:errorcluster, "Wait for Stop?"=w327:bool)  [unwired: 7 in]
            n141 = Merge Errors(w337, w336) -> (w334:errorcluster)
            n142 = call "Error Reported.vi"("Error"=w334, "Module ID"=w323) -> ()  [unwired: 9 in, 1 out]
          }
          frame Default {
            # "'Default' case only runs if there is a message that isn't defined in any of the other cases.  Output a programming error."
            n143 = property on="Property Node" class="Mod Admin"(reference=w348) -> ("Accessors:Module ID"=w347:i32)  [unwired: 1 in, 2 out]
            n144 = call "Module Name--constant.vi"("Module ID"=w347) -> ("Module Name"=w341:string)  [unwired: 10 in]
            n145 = Format Into String(format string="The invalid message string \"%s\" was received in the Message Handling Loop for module \"%s\".", w342, w341) -> (resulting string=w344:string)  [unwired: 2 in, 1 out]
            n146 = call <vilib>:"Error Cluster From Error Code.vi"("show call chain? (False)"=TRUE, "error message (\"\")"=w344, "error code (0)"=1) -> ("error out"=w350:errorcluster)  [unwired: 6 in]
            n147 = Merge Errors(w351, w350) -> (w352:errorcluster)
          }
        }
        n148 = call-dynamic "Delacor_lib_QMH_Error Handler - Message Handling Loop.vi"("error in"=w179, "Message Queue in"=w170) -> ("dup error in"=w176:errorcluster)  [unwired: 8 in, 1 out]
      }
    }
    frame Error {
      n149 = call "Synchronize Caller Events.vi"("Module Admin"=w356) -> ("Module Admin out"=w355:refnum<class "Delacor_lib_QMH_Cloneable Module Admin.lvclass">)  [unwired: 9 in, 1 out]
      n150 = property on="Property Node" class="Mod Admin"(reference=w355) -> ("Accessors:Module ID"=w354:i32)  [unwired: 1 in, 2 out]
      n151 = call-dynamic "Delacor_lib_QMH_Release Message Queue.vi"("error in"=w362, "Message Queue"=w353) -> ("error out"=w361:errorcluster)  [unwired: 9 in]
      n152 = call "Module Name--constant.vi"("Module ID"=w354) -> ("Module Name"=w359:string)  [unwired: 10 in]
      n153 = Format Into String(format string="An error occurred during initialization. %s is no longer running.", w359) -> (resulting string=w357:string)  [unwired: 2 in, 1 out]
      n154 = call "Error Reported.vi"("Additional Information"=w357, "Error"=w361, "Module ID"=w354) -> ()  [unwired: 8 in, 1 out]
    }
  }
  n155 = Merge Errors(w18, w17) -> (w19:errorcluster)
  n156 = call "Close Module.vi"("error in"=w19, "Wait for stop?"=w3, "Module Admin in"=w5) -> ("error out"=w15:errorcluster, "External Launch"=w2:bool, "Module Admin out"=w4:refnum<class "Delacor_lib_QMH_Cloneable Module Admin.lvclass">)  [unwired: 6 in]
  n157 = Unregister For Events(event registration refnum=w10, error in=w15) -> (error out=w14:errorcluster)
  "error out" <- w14
  n158 = case "External Launch?" shown="True" w2 {
    tunnel: w14 -> [_ w363]
    frame False {
    }
    frame True {
      n159 = case shown="No Error" w363 {
        frame No Error {
          n160 = invoke class="VI" method="FP.Close"() -> ()  [unwired: 3 in, 3 out]
        }
        frame Error {
          n161 = disable-structure shown="Default" {
            frame condition #0 (active) {
              n162 = invoke class="VI" method="FP.Open"("Activate"=TRUE ("Activate?")) -> ()  [unwired: 4 in, 5 out]
            }
            frame condition #1 {
              # "Don't show panel on error if running inside a built EXE."
            }
          }
        }
      }
    }
  }
  n163 = local write "Module Admin"(w4) -> ()
